vi "Calculate Plot Range.vi"(8 "error in (no error)":errorcluster, 9 "Coordinates System":enum16{"Cartesian", "Cylindrical", "Spherical"}(ring), 10 "3D Plot Datatype.lvclass in":refnum<class "3D Plot Datatype.lvclass">, 11 "Plot Representation In":T1) -> (0 "error out":errorcluster, 2 "3D Plot Datatype.lvclass out":refnum<class "3D Plot Datatype.lvclass">, 3 "Plot Representation Out":T1)   [LabVIEW 2020, in "3D Plot Datatype.lvclass"]
uses:
  3D Plot Datatype.lvclass
  Plot Representation.ctl
  Range Clusters.ctl
  Mesh Data.ctl
  3D Plot.lvclass
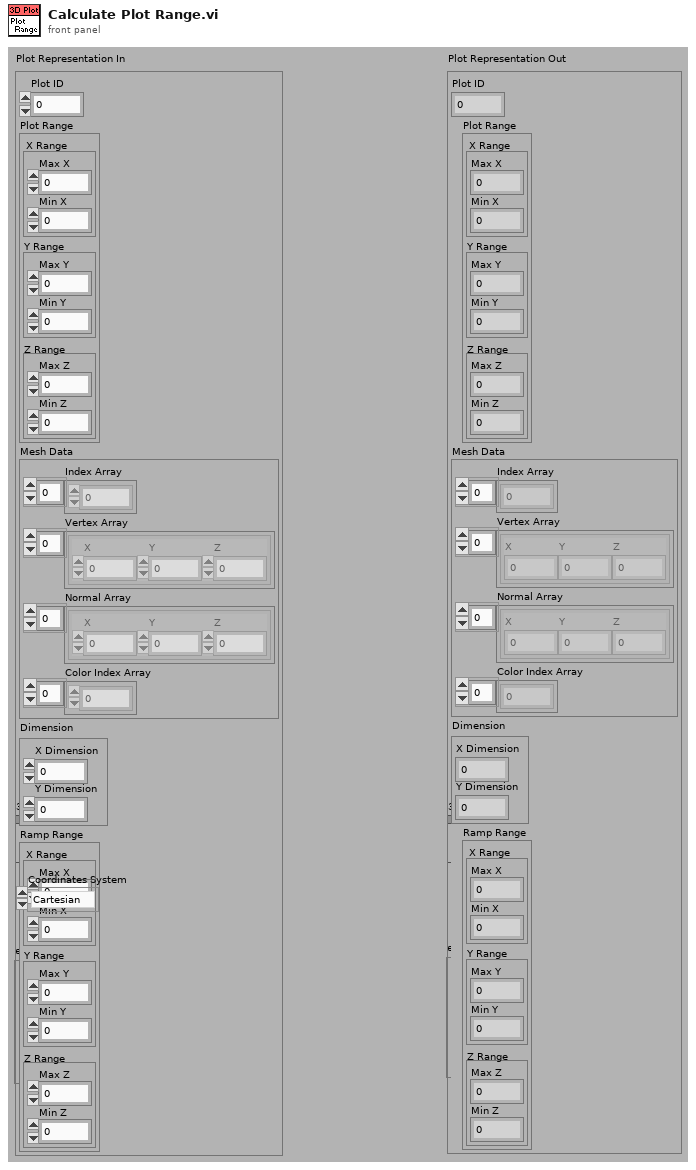
[diagram p1: front panel]
types:
  T1 = typedef "3D Plot.lvclass/Plot Representation.ctl" = cluster{"Plot ID":i32, "Plot Range":T2, "Mesh Data":T3, "Dimension":cluster{"X Dimension":i32, "Y Dimension":i32}, "Ramp Range":T2}
  T2 = typedef "3D Plot.lvclass/Range Clusters.ctl" = cluster{"X Range":cluster{"Max X":sgl, "Min X":sgl}, "Y Range":cluster{"Max Y":sgl, "Min Y":sgl}, "Z Range":cluster{"Max Z":sgl, "Min Z":sgl}}
  T3 = typedef "3D Plot.lvclass/Mesh Data.ctl" = cluster{"Index Array":u32[], "Vertex Array":cluster{"X":sgl, "Y":sgl, "Z":sgl}[], "Normal Array":cluster{"X":sgl, "Y":sgl, "Z":sgl}[], "Color Index Array":i32[]}
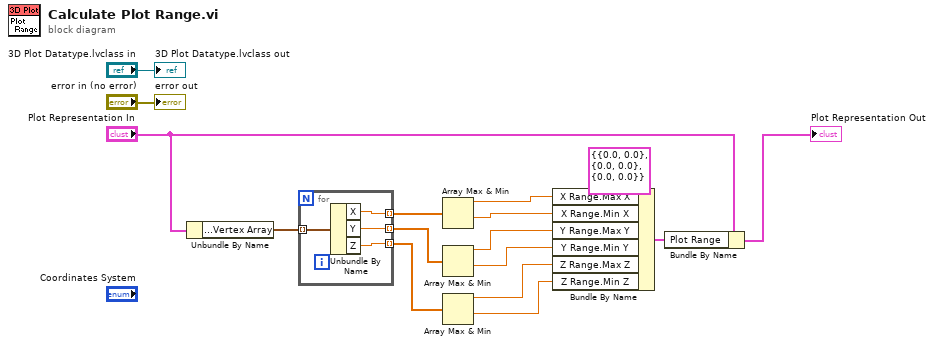
[diagram p0: block diagram]
diagram:
  n1 = Unbundle By Name("Plot Representation In") -> ("Mesh Data.Vertex Array"=w10:cluster{"X":sgl, "Y":sgl, "Z":sgl}[])
  n2 = for {
    tunnel: w10 -> [w20] mode=indexing
    tunnel: [w19] -> w9 mode=indexing
    tunnel: [w18] -> w7 mode=indexing
    tunnel: [w17] -> w8 mode=indexing
    n3 = Unbundle By Name(w20) -> ("X"=w19:sgl, "Y"=w18:sgl, "Z"=w17:sgl)
  }
  n4 = Array Max & Min(array=w9) -> (max value=w6:sgl, min value=w5:sgl)  [unwired: 2 out]
  n5 = Array Max & Min(array=w7) -> (max value=w4:sgl, min value=w3:sgl)  [unwired: 2 out]
  n6 = Array Max & Min(array=w8) -> (max value=w2:sgl, min value=w1:sgl)  [unwired: 2 out]
  n7 = Bundle By Name(cluster=T2 {"X Range"={"Max X"=0.0, "Min X"=0.0}, "Y Range"={"Max Y"=0.0, "Min Y"=0.0}, "Z Range"={"Max Z"=0.0, "Min Z"=0.0}} ("This Range Min/Max Out"), "X Range.Max X"=w6, "X Range.Min X"=w5, "Y Range.Max Y"=w4, "Y Range.Min Y"=w3, "Z Range.Max Z"=w2, "Z Range.Min Z"=w1) -> (w11:T2)
  n8 = Bundle By Name(cluster="Plot Representation In", "Plot Range"=w11) -> (→"Plot Representation Out":T1)
  "error out" <- "error in (no error)"
  "3D Plot Datatype.lvclass out" <- "3D Plot Datatype.lvclass in"
